vi "TCP - Create Rx Transfer.vi"(7 "rx channels":T4[](array[typedef]) {"core"."string offset" format="%d bytes"}, 9 "source address":string="169.254.239.43", 11 "source port":string) -> (8 "Transfer":T1={"core"={"name"="Transfer"}, "component settings"=[], "channels"=[]} {"channels"."core"."string offset" format="%d bytes"})   [LabVIEW 2024]
uses:
  <vilib>/addons/VeriStand Custom Device Scripting APIs/Data Sharing Framework/DSF Core.lvlibp/Typedefs/DSF Engine Channel Configuration.ctl
  <vilib>/addons/VeriStand Custom Device Scripting APIs/Data Sharing Framework/DSF Core.lvlibp/Typedefs/Core Channel Configuration.ctl
  <vilib>/addons/VeriStand Custom Device Scripting APIs/Data Sharing Framework/DSF Core.lvlibp/Typedefs/DSF Data Type.ctl
  <vilib>/addons/VeriStand Custom Device Scripting APIs/Data Sharing Framework/DSF Core.lvlibp/Typedefs/DSF Settings Info.ctl
  <vilib>/addons/VeriStand Custom Device Scripting APIs/Data Sharing Framework/DSF Core.lvlibp/Typedefs/DSF Engine Transfer Configuration.ctl
  <vilib>/addons/VeriStand Custom Device Scripting APIs/Data Sharing Framework/DSF Core.lvlibp/Typedefs/Core Transfer Configuration.ctl
  <vilib>/addons/VeriStand Custom Device Scripting APIs/Data Sharing Framework/DSF Core.lvlibp
  <vilib>/addons/VeriStand Custom Device Scripting APIs/Data Sharing Framework/DSF Core.lvlibp/Classes/Configuration/Core/Channel/Channel Configuration.lvclass
  <vilib>/addons/VeriStand Custom Device Scripting APIs/Data Sharing Framework/DSF Core.lvlibp/Classes/Configuration/Core/Transfer/Transfer Configuration.lvclass
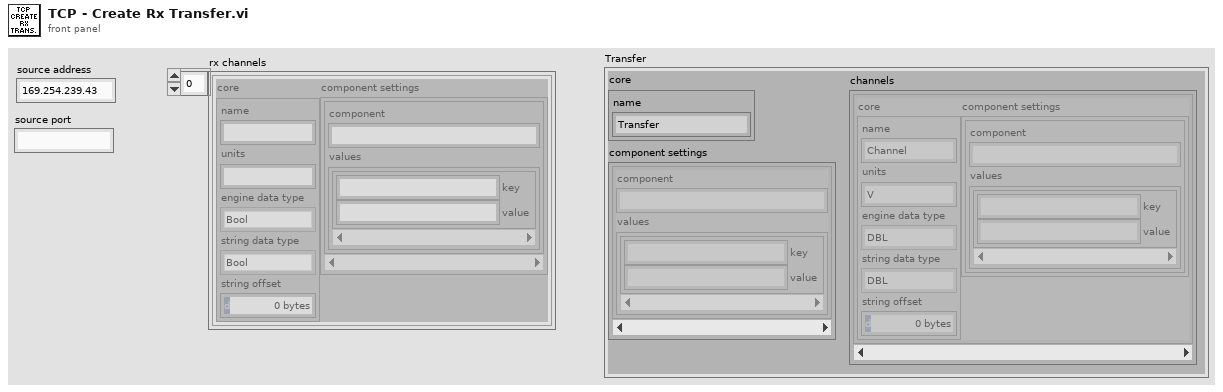
[diagram p1: front panel]
types:
  T1 = typedef "DSF Core.lvlibp/DSF Engine Transfer Configuration.ctl" = cluster{"core":T2, "component settings":T3[], "channels":T4[]}
  T2 = typedef "DSF Core.lvlibp/Transfer Configuration.lvclass/Core Transfer Configuration.ctl" = cluster{"name":string}
  T3 = typedef "DSF Core.lvlibp/DSF Settings Info.ctl" = cluster{"component":string, "values":cluster{"key":string, "value":string}[]}
  T4 = typedef "DSF Core.lvlibp/DSF Engine Channel Configuration.ctl" = cluster{"core":T5, "component settings":T3[]}
  T5 = typedef "DSF Core.lvlibp/Channel Configuration.lvclass/Core Channel Configuration.ctl" = cluster{"name":string, "units":string, "engine data type":T6, "string data type":T6, "string offset":u64}
  T6 = typedef "DSF Core.lvlibp/DSF Data Type.ctl" = enum8{"Bool", "SGL", "DBL", "I8", "I16", "I32", "I64", "U8", "U16", "U32", "U64"}
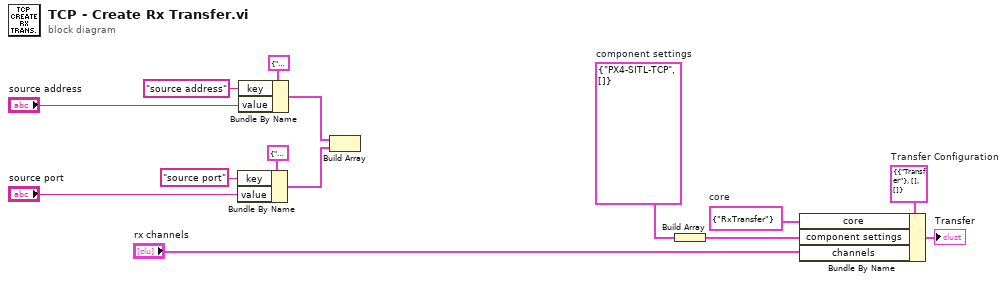
[diagram p0: block diagram]
diagram:
  w1 = T3 {"component"="PX4-SITL-TCP", "values"=[]}  # component settings
  w4 = T2 {"name"="RxTransfer"}  # core
  w5 = T1 {"core"={"name"="Transfer"}, "component settings"=[], "channels"=[]}  # Transfer Configuration
  n1 = Bundle By Name(cluster=cluster{"key":string, "value":string} {"key"="", "value"=""} ("setting"), "key"="source port", "value"="source port") -> (w7:cluster{"key":string, "value":string})
  n2 = Bundle By Name(cluster=cluster{"key":string, "value":string} {"key"="", "value"=""} ("setting"), "key"="source address", "value"="source address") -> (w9:cluster{"key":string, "value":string})
  n3 = Build Array(w9, w7) -> ()  [unwired: 1 out]
  n4 = Build Array(w1) -> (w3:T3[])
  n5 = Bundle By Name(cluster=w5, "core"=w4, "component settings"=w3, "channels"="rx channels") -> (→"Transfer":T1)
